vi "Chronos TDMS Get Plot Names and Limits.vi"(8 "error in (no error)":errorcluster, 11 "Ch Data":T3[](array[typedef])) -> (0 "error out":errorcluster, 3 "Limit Plot Map":T1)   [LabVIEW 2021]
uses:
  Viewer/cluster CC Channel from TDMS.ctl
  GUI/Chronos cluster Map Limit Plots.ctl
  typedefs/Chronos cluster Plot Data and Limits.ctl
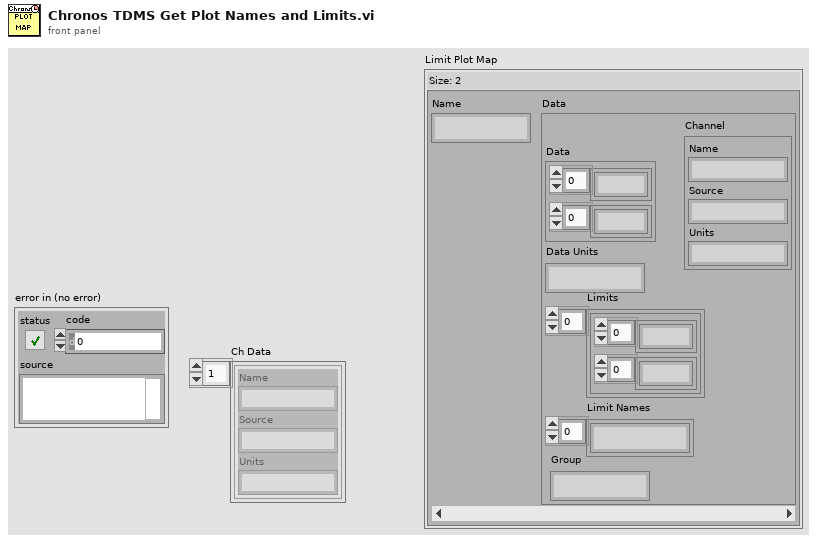
[diagram p1: front panel]
types:
  T1 = typedef "Chronos cluster Map Limit Plots.ctl" = map{string, T2}
  T2 = typedef "Chronos cluster Plot Data and Limits.ctl" = cluster{"Data":cluster{dbl[], dbl[]}, "Data Units":string, "Limits":cluster{dbl[], dbl[]}[], "Limit Names":string[], "Channel":T3, "Group":string}
  T3 = typedef "cluster CC Channel from TDMS.ctl" = cluster{"Name":string, "Source":string, "Units":string}
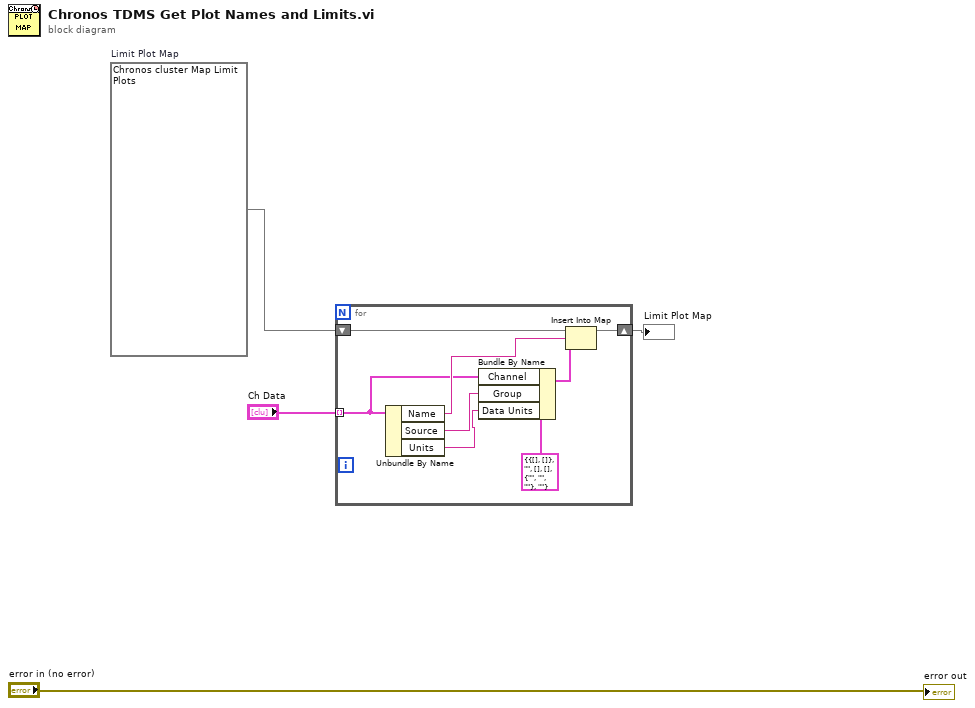
[diagram p0: block diagram]
diagram:
  w3 = T1 {}  # Limit Plot Map
  n1 = for {
    tunnel: "Ch Data" -> [w6] mode=indexing
    shift-right: [w11] -> w1
    shift-left: w3 -> [w12]
    n2 = Unbundle By Name(w6) -> ("Name"=w7:string, "Source"=w9:string, "Units"=w5:string)
    n3 = Bundle By Name(cluster=T2 {"Data"={[], []}, "Data Units"="", "Limits"=[], "Limit Names"=[], "Channel"={"Name"="", "Source"="", "Units"=""}, "Group"=""} ("Data"), "Channel"=w6, "Group"=w9, "Data Units"=w5) -> (w8:T2)
    n4 = Insert Into Map(map in=w12, key=w7, value=w8) -> (map out=w11:T1)  [unwired: 2 out]
  }
  "Limit Plot Map" <- w1
  "error out" <- "error in (no error)"
